vi "UpdateValue.vi"(7 "Qbus in":refnum<class "Qbus.lvclass">, 8 "error in (no error)":errorcluster, 10 "Numeric":dbl, 11 "channel":T1) -> (0 "error out":errorcluster)   [LabVIEW 2017, in "ModbusMaster.lvlib"]
uses:
  <vilib>/addons/InsightCM/Devices/Shared/Common/ModbusMaster/ModbusMaster.lvlib
  <vilib>/addons/Qbus/Qbus.lvclass
  <vilib>/addons/InsightCM/Devices/Shared/Common/ModbusMaster/controls/ModbusChannel.ctl
  <vilib>/addons/InsightCM/Devices/Shared/Common/ModbusMaster/controls/RegisterType.ctl
  <vilib>/addons/PointValueMap/subVIs/Point_Write_double.vi
  <vilib>/addons/PointValueMap/PointValueMap.lvlib
  <vilib>/addons/InsightCM/Utilities/ChannelStatus/ChannelStatus.lvlib
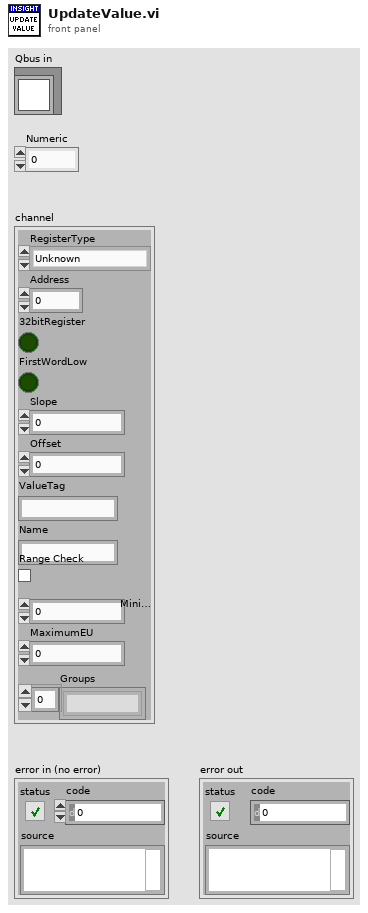
[diagram p1: front panel]
types:
  T1 = typedef "ModbusMaster.lvlib/ModbusChannel.ctl" = cluster{"RegisterType":T2, "Address":i32, "32bitRegister":bool, "FirstWordLow":bool, "Slope":dbl, "Offset":dbl, "ValueTag":string, "Name":string, "Range Check":bool, "MinimumEU":dbl, "MaximumEU":dbl, "Groups":string[]}
  T2 = typedef "ModbusMaster.lvlib/RegisterType.ctl" = enum16{"Unknown", "Coil", "Discrete Input", "Holding Register", "Input Register"}
  T3 = typedef "PointValueMap.lvlib/PointMap.ctl" = refnum<data-value>
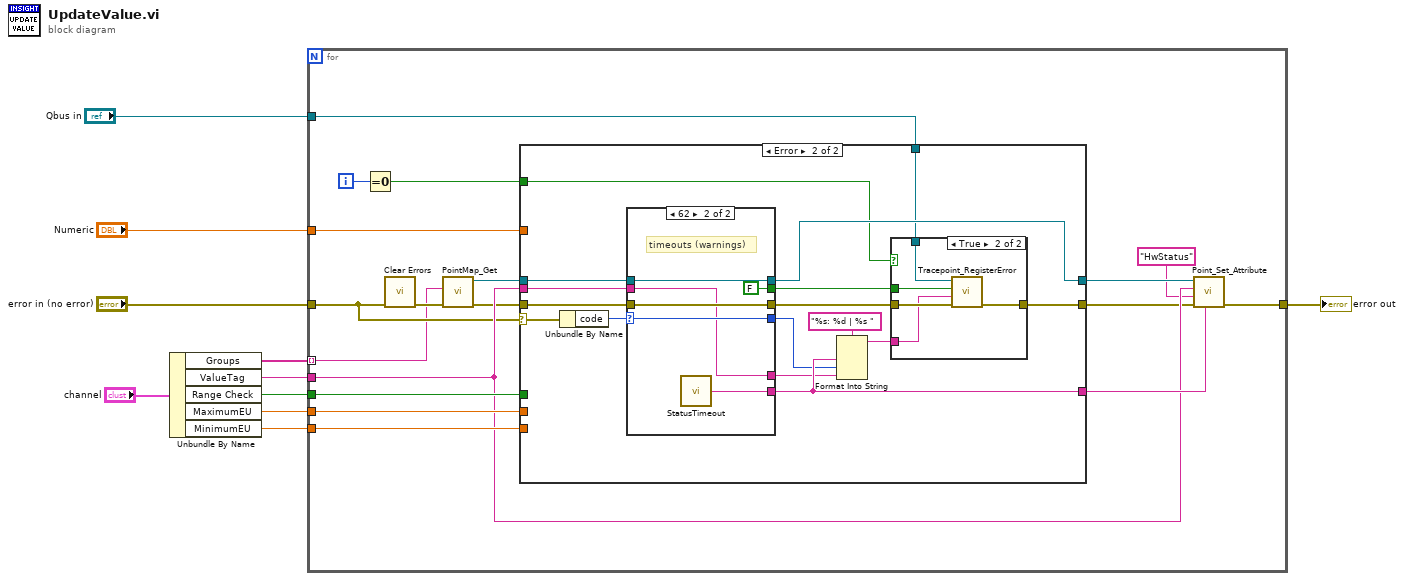
[diagram p0: block diagram]
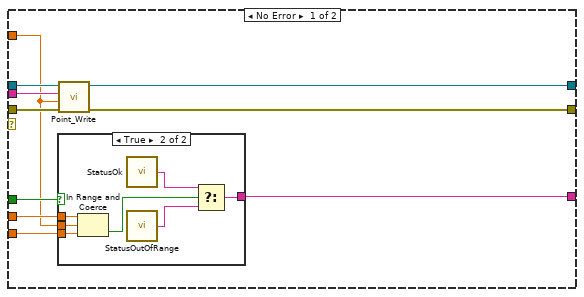
[diagram p2: hidden frame]
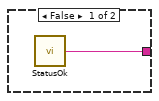
[diagram p3: hidden frame]
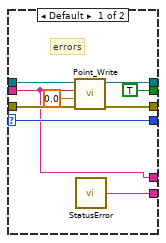
[diagram p5: hidden frame]
diagram:
  n1 = Unbundle By Name("channel") -> ("Groups"=w1:string[], "ValueTag"=w5:string, "Range Check"=w6:bool, "MaximumEU"=w8:dbl, "MinimumEU"=w9:dbl)
  n2 = for {
    tunnel: "Qbus in" -> [w28]
    tunnel: w9 -> [w26]
    tunnel: w8 -> [w25]
    tunnel: w6 -> [w24]
    tunnel: w5 -> [w23]
    tunnel: "Numeric" -> [w16]
    tunnel: w1 -> [w13] mode=indexing
    tunnel: "error in (no error)" -> [w17]
    tunnel: [w22] -> w4
    i -> [w12]
    n3 = Equal To 0?(x=w12) -> (x = 0?=w11:bool)
    n4 = call <vilib>:"Clear Errors.vi"("error in (no error)"=w17) -> ("error out"=w18:errorcluster)  [unwired: 5 in, 1 out]
    n5 = call <vilib>:"PointMap_Get.vi"("error in (no error)"=w18, "Name"=w13) -> ("error out"=w14:errorcluster, "Map Out"=w15:T3)  [unwired: 7 in, 1 out]
    n6 = case shown="Error" w17 {
      selector: w17 -> [_ w61]
      tunnel: w14 -> [w38 w60]
      tunnel: w15 -> [w37 w58]
      tunnel: w23 -> [w34 w57]
      tunnel: w16 -> [w30 _]
      tunnel: [w35 w55] -> w21
      tunnel: [w36 w59] -> w20
      tunnel: [w29 w51] -> w27
      tunnel: w24 -> [w33 _]
      tunnel: w25 -> [w31 _]
      tunnel: w26 -> [w32 _]
      tunnel: w28 -> [_ w54]
      tunnel: w11 -> [_ w47]
      frame No Error {
        n7 = case shown="True" w33 {
          tunnel: w32 -> [_ w45]
          tunnel: w31 -> [_ w46]
          tunnel: w30 -> [_ w44]
          tunnel: [w39 w42] -> w29
          frame False {
            n8 = call <vilib>:"StatusOk.vi"() -> ("status"=w39:string)  [unwired: 5 in]
          }
          frame True {
            n9 = In Range and Coerce(upper limit=w46, x=w44, lower limit=w45) -> (In Range?=w43:bool)  [unwired: 1 out]
            n10 = call <vilib>:"StatusOk.vi"() -> ("status"=w41:string)  [unwired: 5 in]
            n11 = call <vilib>:"StatusOutOfRange.vi"() -> ("status"=w40:string)  [unwired: 5 in]
            n12 = Select(t=w41, s=w43, f=w40) -> (s? t:f=w42:string)
          }
        }
        n13 = call-poly <vilib>:"Point_Write.vi"("Error In"=w38, "Value"=w30, "Tag"=w34, "Map"=w37) -> ("Error Out"=w35:errorcluster, "Map Out"=w36:T3)  [unwired: 6 in]
      }
      frame Error {
        n14 = Unbundle By Name(w61) -> ("code"=w52:i32)
        n15 = case shown="62" w52 {
          selector: w52 -> [w71 w81]
          tunnel: [w74 w83] -> w56
          tunnel: w60 -> [w76 w83]
          tunnel: [w75 w82] -> w59
          tunnel: w58 -> [w77 w82]
          tunnel: w57 -> [w70 w79]
          tunnel: [w72 w80] -> w51
          tunnel: [w71 w81] -> w50
          tunnel: [w70 w79] -> w49
          tunnel: [TRUE ("Error") FALSE ("Error")] -> w48
          frame Default {
            # "errors"
            n16 = call-poly <vilib>:"Point_Write.vi"("Error In"=w76, "Value"=0.0, "Tag"=w70, "Map"=w77) -> ("Error Out"=w74:errorcluster, "Map Out"=w75:T3)  [unwired: 6 in]
            n17 = call <vilib>:"StatusError.vi"() -> ("status"=w72:string)  [unwired: 5 in]
          }
          frame 62 {
            # "timeouts (warnings)"
            n18 = call <vilib>:"StatusTimeout.vi"() -> ("status"=w80:string)  [unwired: 5 in]
          }
        }
        n19 = Format Into String(format string="%s: %d | %s ", w51, w50, w49) -> (resulting string=w53:string)  [unwired: 2 in, 1 out]
        n20 = case shown="True" w47 {
          tunnel: w56 -> [w63 w68]
          tunnel: [w63 w67] -> w55
          tunnel: w54 -> [_ w66]
          tunnel: w53 -> [_ w65]
          tunnel: w48 -> [_ w64]
          frame False {
          }
          frame True {
            n21 = call <vilib>:"Tracepoint_RegisterError.vi"("error in (no error)"=w68, "log string"=w65, "Error"=w64, "Qbus"=w66) -> ("error out"=w67:errorcluster)  [unwired: 7 in]
          }
        }
      }
    }
    n22 = call <vilib>:"Point_Set_Attribute.vi"("Value"=w27, "Error In"=w21, "Attribute"="HwStatus", "Tag"=w23, "Map"=w20) -> ("Error Out"=w22:errorcluster)  [unwired: 5 in, 1 out]
  }
  "error out" <- w4
